vi "ZMC Make One File Zpj.vi"(8 "error in (no error)":errorcluster caption="错误输入（无错误）", 9 "pBasfilename":string, 10 "pBasDir":string, 11 "pZpjBuff":u32) -> (0 "error out":errorcluster caption="错误输出", 1 "function return":i32, 2 "pBasDir out":string, 3 "pZpjBuff out":u32)   [LabVIEW 2015, in "zauxdll.lvlib"]
doc: "int32 __stdcall ZMC_MakeOneFileZpj(void *pZpjBuff, char *pBasDir, const char* pBasfilename);"
uses:
  zauxdll.lvlib
  zmotion.dll
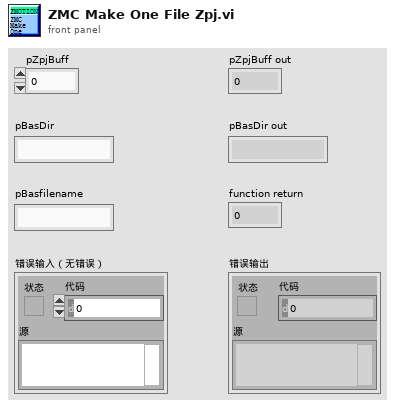
[diagram p1: front panel]
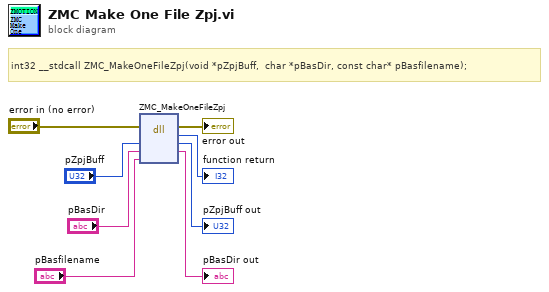
[diagram p0: block diagram]
diagram:
  # "int32 __stdcall ZMC_MakeOneFileZpj(void *pZpjBuff,  char *pBasDir, const char* pBasfilename);"
  n1 = dll-call lib="C:/Users/VIC/Desktop/GOGORO_SA/system/LLB/zmotion/zaux/zmotion.*" fn="ZMC_MakeOneFileZpj"(error in="error in (no error)", "pZpjBuff"="pZpjBuff", "pBasDir"="pBasDir", "pBasfilename"="pBasfilename") -> (error out=→"error out":errorcluster, →"function return":i32, "pZpjBuff"=→"pZpjBuff out":u32, "pBasDir"=→"pBasDir out":string)  [unwired: 3 in, 1 out]
